vi "Read Batch Data value.vi"(8 "error in (no error)":errorcluster, 11 "Domino Laser module Class in":refnum<class "Domino Laser module Class.lvclass">) -> (0 "error out":errorcluster, 2 "Batch Data":T1, 3 "Domino Laser module Class out":refnum<class "Domino Laser module Class.lvclass">)   [LabVIEW 2015, in "Domino LM.lvlib" / "Domino Laser module Class.lvclass"]
uses:
  CTRLS/Domino Laser module Class.lvclass
  CTRLS/Open Batch Data.ctl
  CTRLS/Domino Laser module Class.lvclass/Domino Laser module Class.ctl
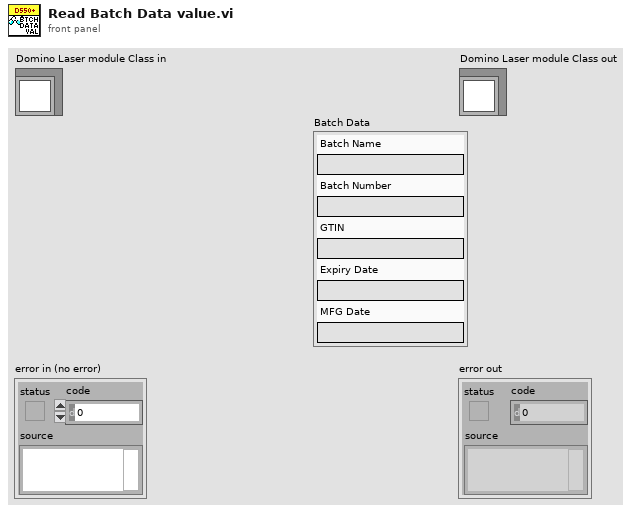
[diagram p1: front panel]
types:
  T1 = typedef "Open Batch Data.ctl" = cluster{"Batch Name":string, "Batch Number":string, "GTIN":string, "Expiry Date":string, "MFG Date":string}
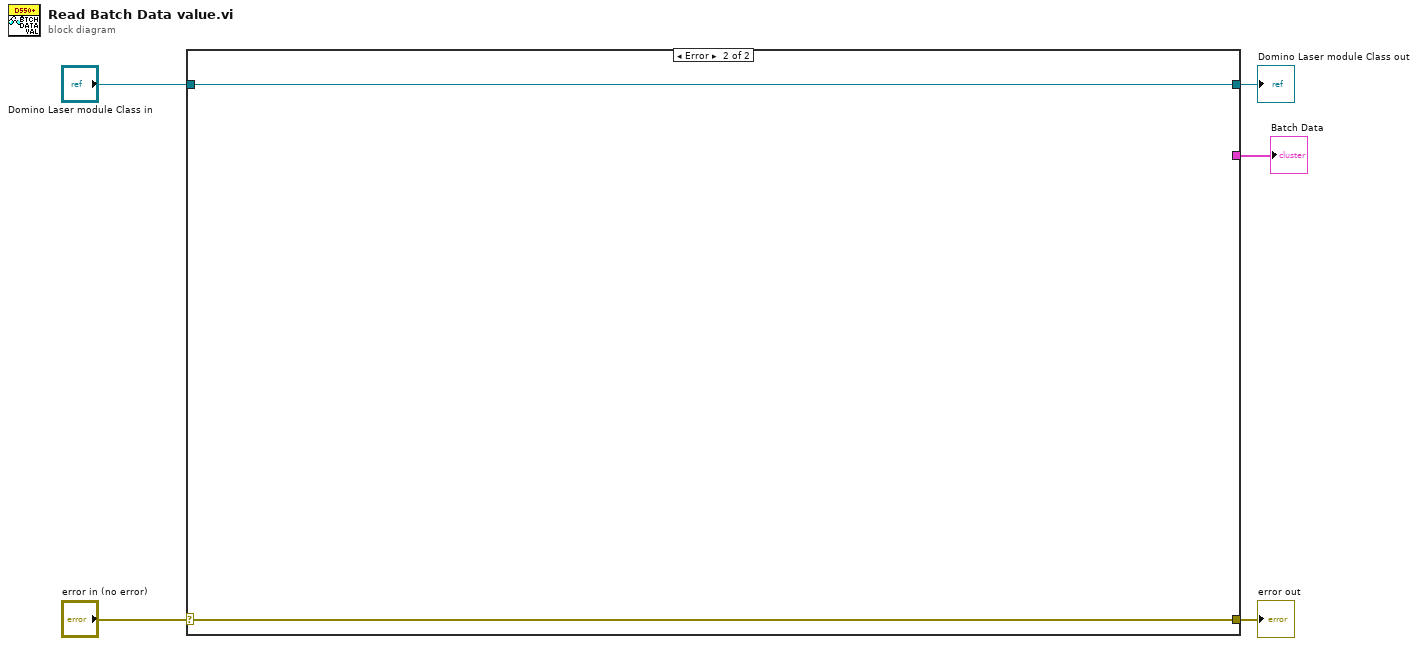
[diagram p0: block diagram]
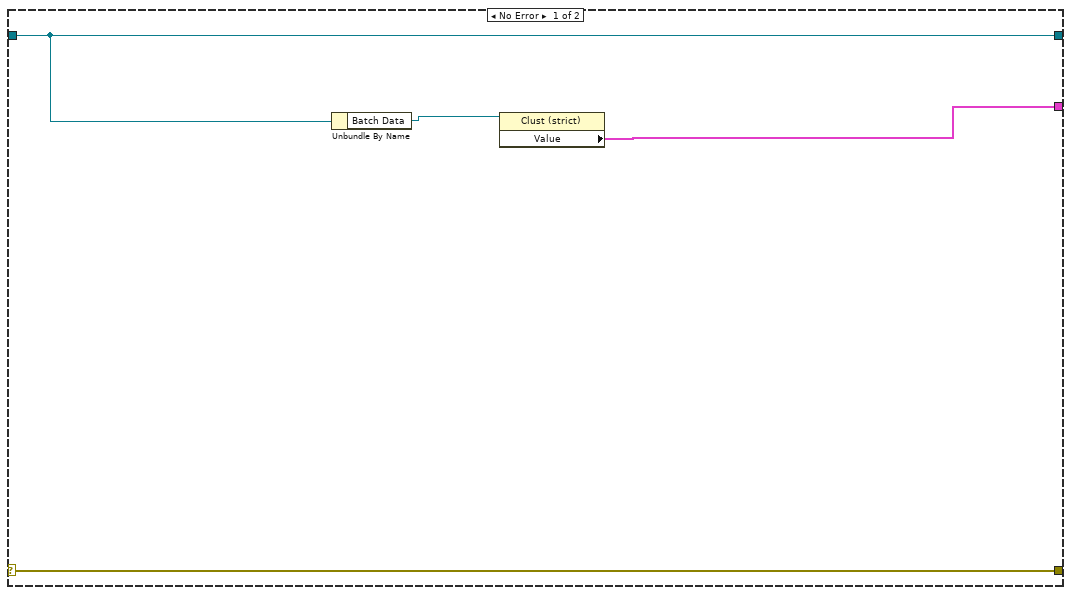
[diagram p2: hidden frame]
diagram:
  n1 = case shown="Error" "error in (no error)" {
    selector: "error in (no error)" -> [w9 w10]
    tunnel: [w9 w10] -> w4
    tunnel: [w8 w11] -> w2
    tunnel: "Domino Laser module Class in" -> [w8 w11]
    tunnel: [w6 _] -> w1
    frame No Error {
      n2 = Unbundle By Name(w8) -> ("Batch Data"=w7:refnum<vi>)
      n3 = property class="Clust (strict)"(reference=w7) -> ("Value"=w6:T1)  [unwired: 1 in, 2 out]
    }
    frame Error {
    }
  }
  "error out" <- w4
  "Domino Laser module Class out" <- w2
  "Batch Data" <- w1
